vi "MGCC_Global_communication_inputsettings .vi"() -> ()   [LabVIEW 2016]
panel:
  in  "Digital control channel number PV":dbl
  in  "Digital statues channel number PV":dbl
  in  "Analogue control channel number PV":dbl
  in  "Analogue statues channel number PV":dbl
  in  "DNP3 Outstation Address PV":dbl
  in  "DNP3 Master Address PV":dbl
  in  "DNP3 port PV":dbl
  in  "IP_PV":dbl[](array[numeric])
  in  "Digital control channel number BESS":dbl
  in  "Digital statues channel number BESS":dbl
  in  "Analogue control channel number BESS":dbl
  in  "Analogue statues channel number BESS":dbl
  in  "DNP3 Outstation Address BESS":dbl
  in  "DNP3 Master Address BESS":dbl
  in  "DNP3 port BESS":dbl
  in  "IP_BESS":dbl[](array[numeric])
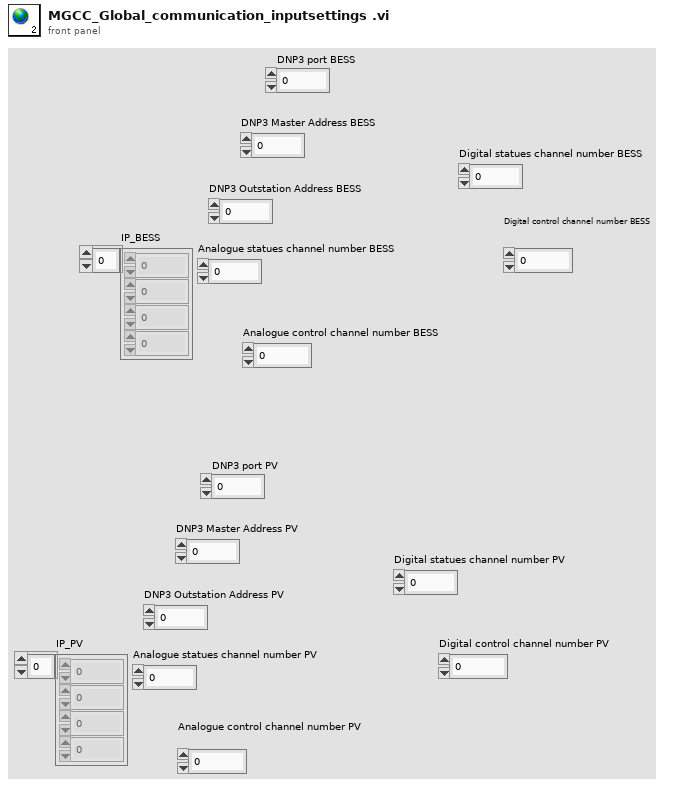
[diagram p1: front panel]
diagram:
